vi "wfm_feature init.vi"(6 "signalDataAttr":T1, 8 "error in (no error)":errorcluster, 10 "refnum cluster input":T2, 11 "wfm_feature in":refnum<class "wfm_feature.lvclass">) -> (0 "error out":errorcluster, 3 "wfm_feature out":refnum<class "wfm_feature.lvclass">)   [LabVIEW 2018, in "wfm_feature.lvclass"]
uses:
  wfm_feature.lvclass
  PublicSubVI/Class/Sig2MS/ctl/signalDataAttr.ctl
  wfm_feature.lvclass/wfm_feature.ctl
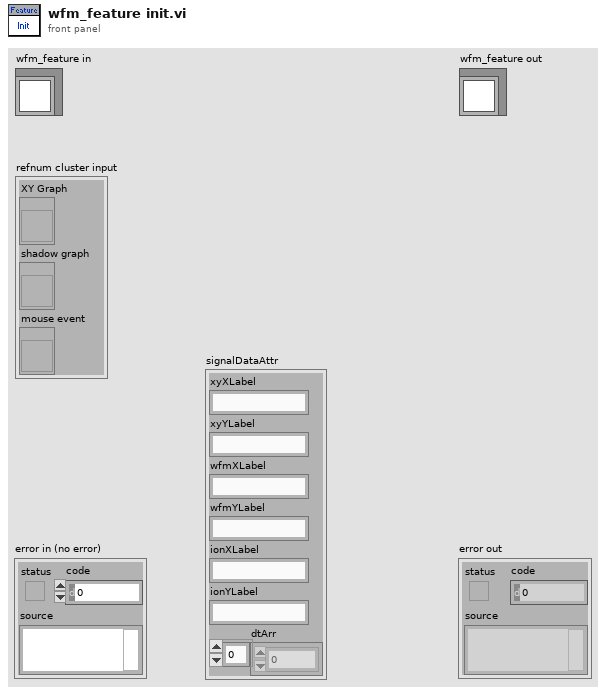
[diagram p1: front panel]
types:
  T1 = typedef "signalDataAttr.ctl" = cluster{"xyXLabel":string, "xyYLabel":string, "wfmXLabel":string, "wfmYLabel":string, "ionXLabel":string, "ionYLabel":string, "dtArr":dbl[]}
  T2 = cluster{"XY Graph":refnum<vi>, "shadow graph":refnum<vi>, "mouse event":refnum<vi>}
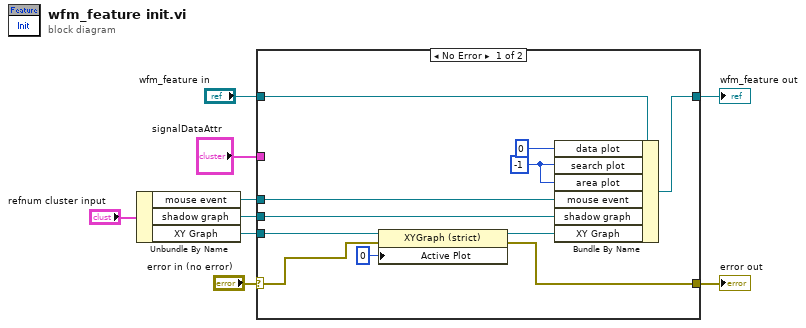
[diagram p0: block diagram]
diagram:
  n1 = Unbundle By Name("refnum cluster input") -> ("mouse event"=w5:refnum<vi>, "shadow graph"=w3:refnum<vi>, "XY Graph"=w4:refnum<vi>)
  n2 = case shown="No Error" "error in (no error)" {
    selector: "error in (no error)" -> [w10 w22]
    tunnel: w4 -> [w11 _]
    tunnel: "wfm_feature in" -> [w20 w21]
    tunnel: [w17 w21] -> w7
    tunnel: [w14 w22] -> w6
    tunnel: w5 -> [w16 _]
    tunnel: w3 -> [w15 _]
    tunnel: "signalDataAttr" -> [_ _]
    frame No Error {
      w12 = -1 ("threshold plot")
      n3 = property class="XYGraph (strict)"(reference=w11, error in=w10, "Active Plot"=u32 0) -> (reference out=w18:refnum<vi>, error out=w14:errorcluster)
      n4 = Bundle By Name(cluster=w20, "data plot"=0 ("Active Plot"), "search plot"=w12, "area plot"=w12, "mouse event"=w16, "shadow graph"=w15, "XY Graph"=w18) -> (w17:refnum<class "wfm_feature.lvclass">)
    }
    frame Error {
    }
  }
  "error out" <- w6
  "wfm_feature out" <- w7
